vi "ReadConfig.vi"(8 "error in (no error)":errorcluster) -> (0 "error out":errorcluster, 3 "Config":T1={"Path"="C:\\Glass", "Days to Keep"=30, "Number of Rows"=90})   [LabVIEW 2015, in "ConfigHelper.lvlib"]
uses:
  ConfigHelper.lvlib
  Config.ctl
  <vilib>/addons/PointValueMap/subVIs/Point_Write_variant.vi
  <vilib>/addons/PointValueMap/PointValueMap.lvlib
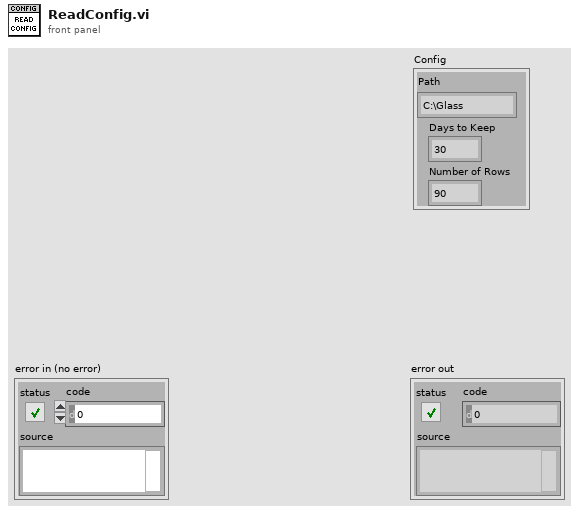
[diagram p1: front panel]
types:
  T1 = typedef "ConfigHelper.lvlib/Config.ctl" = cluster{"Path":string, "Days to Keep":i32, "Number of Rows":i32}
  T2 = typedef "PointValueMap.lvlib/PointMap.ctl" = refnum<data-value>
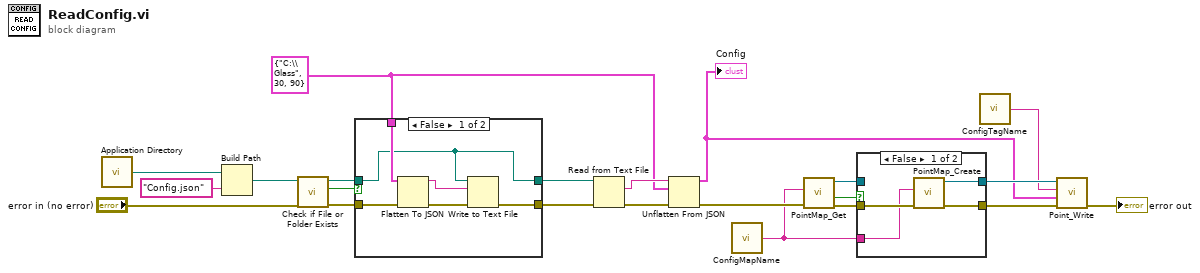
[diagram p0: block diagram]
diagram:
  w12 = T1 {"Path"="C:\\Glass", "Days to Keep"=30, "Number of Rows"=90} ("Config")
  n1 = call <vilib>:"Application Directory.vi"() -> ("Application Directory"=w22:path)
  n2 = Build Path(base path=w22, name or relative path="Config.json") -> (appended path=w20:path)
  n3 = call <vilib>:"Check if File or Folder Exists.vi"("error in (no error)"="error in (no error)", "path"=w20) -> ("error out"=w17:errorcluster, "file or folder exists?"=w19:bool, "dup path"=w18:path)  [unwired: 7 in]
  n4 = case shown="False" w19 {
    tunnel: w18 -> [w23 w30]
    tunnel: w17 -> [w28 w29]
    tunnel: [w26 w29] -> w15
    tunnel: w12 -> [w25 _]
    tunnel: [w23 w30] -> w16
    frame False {
      n5 = Flatten To JSON(anything=w25, error in (no error)=w28) -> (JSON string=w24:string, 11:w27:errorcluster)  [unwired: 1 in]
      n6 = Write to Text File(file (use dialog)=w23, text=w24, error in=w27) -> (error out=w26:errorcluster)  [unwired: 1 in, 2 out]
    }
    frame True {
    }
  }
  n7 = Read from Text File(file (use dialog)=w16, error in=w15) -> (text=w13:string, error out=w14:errorcluster)  [unwired: 2 in, 2 out]
  n8 = Unflatten From JSON(JSON string=w13, type and defaults=w12, error in (no error)=w14) -> (value=w5:T1, error out=w11:errorcluster)  [unwired: 4 in]
  "Config" <- w5
  n9 = call "ConfigMapName.vi"() -> ("Name"=w4:string)  [unwired: 5 in]
  n10 = call <vilib>:"PointMap_Get.vi"("error in (no error)"=w11, "Name"=w4) -> ("error out"=w9:errorcluster, "Found?"=w10:bool, "Map Out"=w8:T2)  [unwired: 7 in]
  n11 = case shown="False" w10 {
    tunnel: w9 -> [w34 w35]
    tunnel: w8 -> [_ w36]
    tunnel: w4 -> [w33 _]
    tunnel: [w32 w36] -> w6
    tunnel: [w31 w35] -> w7
    frame False {
      n12 = call <vilib>:"PointMap_Create.vi"("error in (no error)"=w34, "Name"=w33) -> ("error out"=w31:errorcluster, "Map Out"=w32:T2)  [unwired: 8 in]
    }
    frame True {
    }
  }
  n13 = call "ConfigTagName.vi"() -> ("Name"=w3:string)  [unwired: 5 in]
  n14 = call-poly <vilib>:"Point_Write.vi"("Error In"=w7, "Value"=w5, "Tag"=w3, "Map"=w6) -> ("Error Out"=→"error out":errorcluster)  [unwired: 6 in, 1 out]
